vi "Get Peak Frequency and Amplitude.vi"(10 "IQ Rate (S/s)":dbl, 11 "Power Spectrum / PSD (dBm)":cluster{"f0":dbl, "df":dbl, "magnitude":dbl[]}) -> (2 "Peak Frequency":dbl, 3 "Peak Amplitude":dbl)   [LabVIEW 2017]
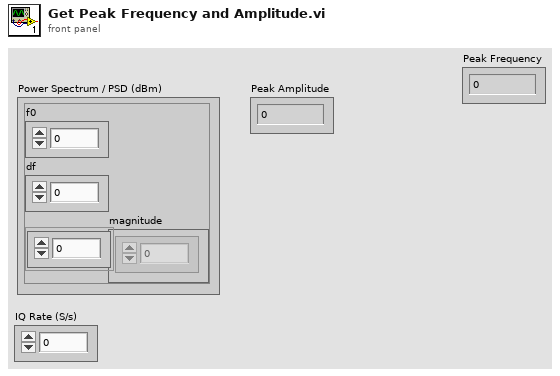
[diagram p1: front panel]
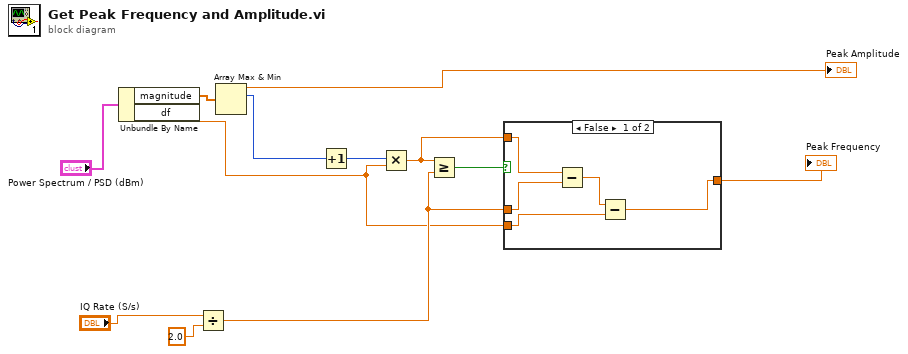
[diagram p0: block diagram]
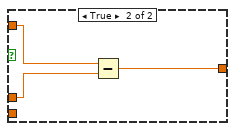
[diagram p2: hidden frame]
diagram:
  n1 = Unbundle By Name("Power Spectrum / PSD (dBm)") -> ("magnitude"=w11:dbl[], "df"=w1:dbl)
  n2 = Divide(x="IQ Rate (S/s)", y=2.0) -> (x/y=w4:dbl)
  n3 = Array Max & Min(array=w11) -> (max value=→"Peak Amplitude":dbl, max index (indices)=w5:i32)  [unwired: 2 out]
  n4 = Increment(x=w5) -> (x+1=w7:i32)
  n5 = Multiply(x=w7, y=w1) -> (x*y=w3:dbl)
  n6 = Greater Or Equal?(x=w3, y=w4) -> (x >= y?=w6:bool)
  n7 = case shown="False" w6 {
    tunnel: w4 -> [w16 w19]
    tunnel: w3 -> [w17 w20]
    tunnel: [w13 w18] -> w2
    tunnel: w1 -> [w15 _]
    frame False {
      n8 = Subtract(x=w17, y=w16) -> (x-y=w14:dbl)
      n9 = Subtract(x=w14, y=w15) -> (x-y=w13:dbl)
    }
    frame True {
      n10 = Subtract(x=w20, y=w19) -> (x-y=w18:dbl)
    }
  }
  "Peak Frequency" <- w2
